vi "prueba.vi"() -> ()   [LabVIEW 2024]
panel:
  out "Measures Plot":dbl[][](graph)
  in  "min_threshold":dbl=5.0 format="%#_13g"
  in  "tolerance%":dbl=4.0 format="%#_13g"
  out "average":dbl
  out "close_values":dbl[](array[numeric]) format="%.2f"
  out "num_elements_found":i32
  out "close_values_w_zeros":dbl[](array[numeric]) format="%.2f"
  in  "data":dbl[](array[numeric])=[0.0, 0.0, 1.0, 2.0, 3.0, 9.3, 9.4, 9.5, 9.4, 9.2, 9.1, 5.0, 4.5, 4.0, 3.0, 2.0, 1.0, 0.0, 0.0] format="%.2f"
  in  "module path":path=path "C:/Users/Taboada.r248/Documents/LabVIEW Projects/LabVIEW-2024-and-Python/pyhthon_modules/find_consecutive_close_values.py"
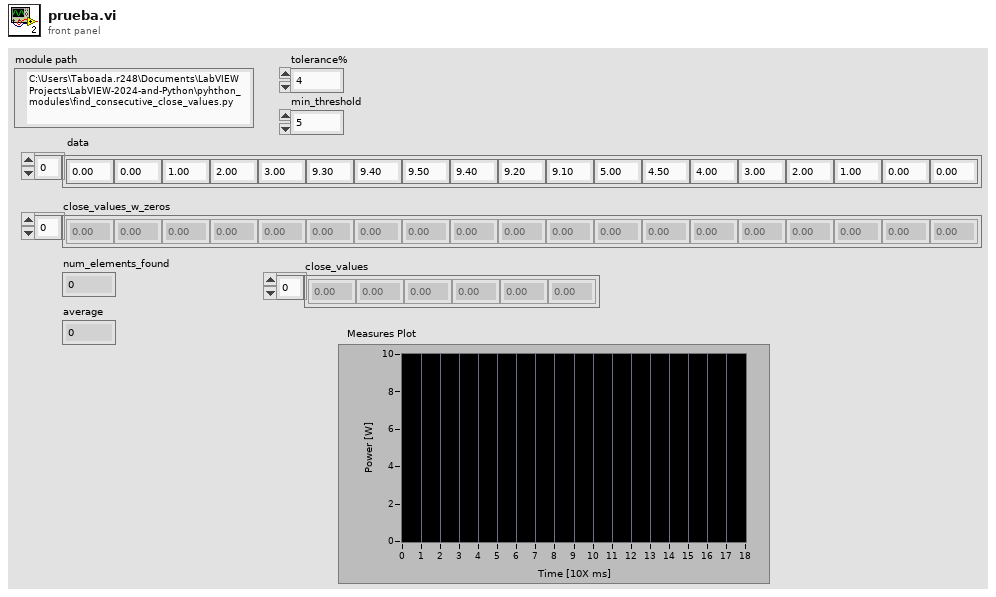
[diagram p1: front panel]
types:
  T1 = cluster{"close_values_w_zeros":dbl[], "num_elements_found":i32, "close_values":dbl[], "average":dbl}
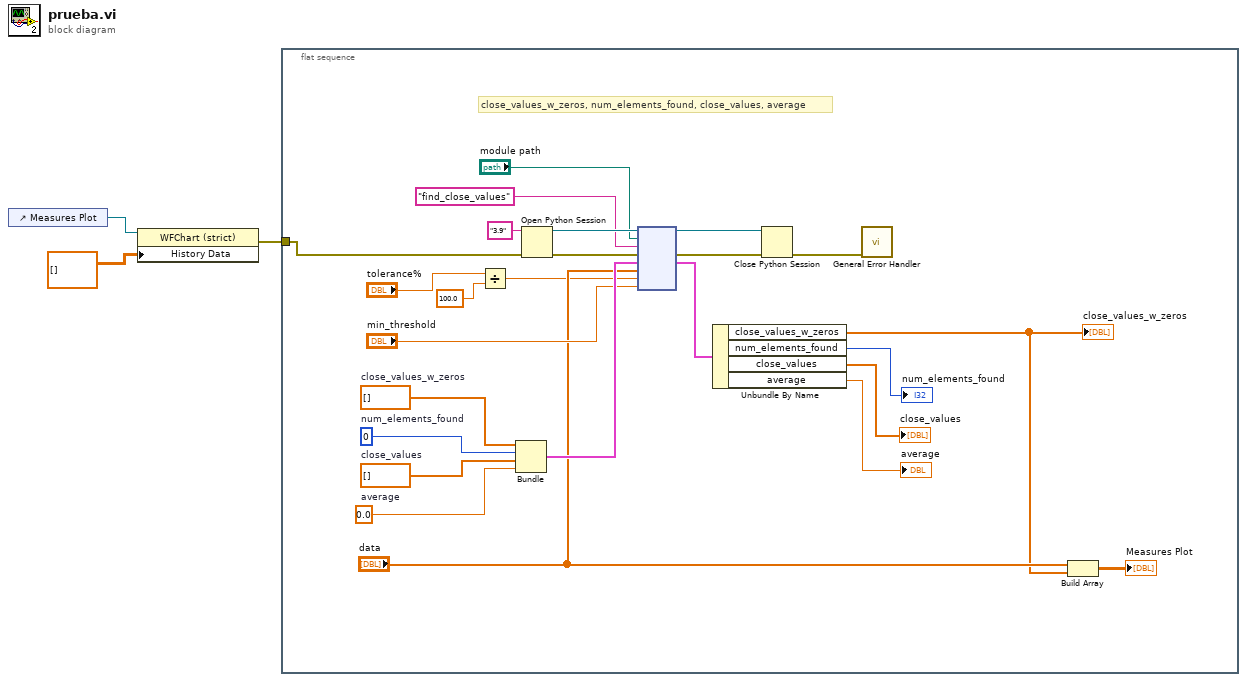
[diagram p0: block diagram]
diagram:
  n1 = control-ref of="Measures Plot"() -> (w3:refnum<vi>)
  n2 = property class="WFChart (strict)"(reference=w3, "History Data"=dbl[][] []) -> (error out=w1:errorcluster)  [unwired: 1 in, 1 out]
  n3 = flat-sequence {
    tunnel: w1 -> [w8]
    frame #0 {
      w17 = 0.0  # average
      w18 = dbl[] []  # close_values
      w19 = 0  # num_elements_found
      w20 = dbl[] []  # close_values_w_zeros
      # "close_values_w_zeros, num_elements_found, close_values, average"
      n4 = Divide(x="tolerance%", y=100.0) -> (x/y=w4:dbl)
      n5 = Bundle("close_values_w_zeros"=w20, "num_elements_found"=w19, "close_values"=w18, "average"=w17) -> (w16:T1)  [unwired: 1 in]
      n6 = Open Python Session(python version="3.9" ("Python version"), 3:w8) -> (session out=w25:refnum<k35>, error out=w28:errorcluster)  [unwired: 1 in]
      n7 = node(w25, "module path", "find_close_values" ("function name"), w28, w16, "data", w4, "min_threshold") -> (w24:refnum<k35>, w27:errorcluster, w14:T1)  [unwired: 3 in, 2 out]
      n8 = Unbundle By Name(w14) -> ("close_values_w_zeros"=w7:dbl[], "num_elements_found"=→"num_elements_found":i32, "close_values"=→"close_values":dbl[], "average"=→"average":dbl)
      "close_values_w_zeros" <- w7
      n9 = Close Python Session(session in=w24, error in=w27) -> (11:w23:errorcluster)
      n10 = call <vilib>:"General Error Handler.vi"("error in (no error)"=w23) -> ()  [unwired: 10 in, 5 out]
      n11 = Build Array("data", w7) -> (→"Measures Plot":dbl[][])
    }
  }
